vi "Start Live View.vi"(8 "error in (no error)":errorcluster, 10 "Camera State In":T3 {"Sub Region"."V Size"."Value" min=0 max=0 step=4; "Sub Region"."H Size"."Value" min=0 max=0 step=4; "Sub Region"."V Offset"."Value" min=0 max=0 step=4; "Sub Region"."H Offset"."Value" min=0 max=0 step=4}, 11 "Acquisition Settings":T1={"Save?"=FALSE, "DCIMG Path"=path "E:/test2", "Filename"="test", "Total Frames"=15, "Sender"=enum."UI"}) -> (0 "error out":errorcluster {"code" format="%.0x"}, 1 "New Image Out":T2, 2 "Camera State Out":T3 {"Sub Region"."V Size"."Value" min=0 max=0 step=4; "Sub Region"."H Size"."Value" min=0 max=0 step=4; "Sub Region"."V Offset"."Value" min=0 max=0 step=4; "Sub Region"."H Offset"."Value" min=0 max=0 step=4})   [LabVIEW 2015, in "Camera.lvlib"]
uses:
  Camera.lvlib
  Camera State.ctl
  Camera Loop State.ctl
  <vilib>/Utility/miscctls.llb/LVMinMaxIncTypeDef.ctl
  Acquisition Settings.ctl
  Live View State.ctl
  <vilib>/vision/Image Controls.llb/IMAQ Image.ctl
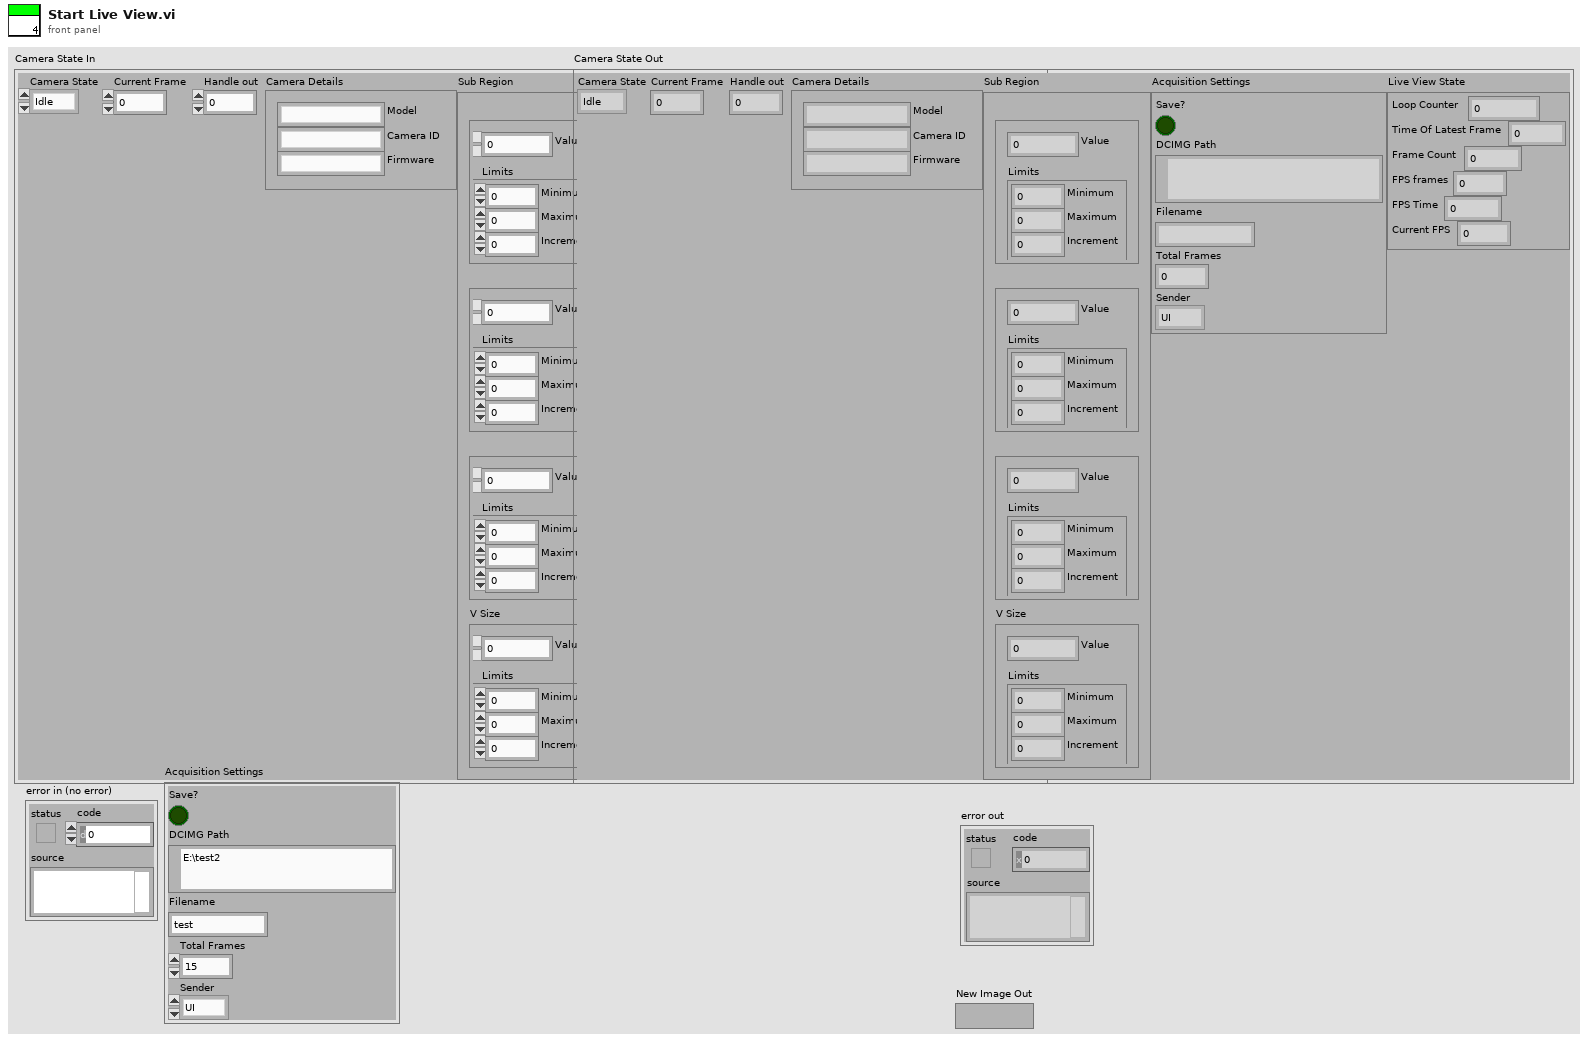
[diagram p1: front panel]
types:
  T1 = typedef "Camera.lvlib/Acquisition Settings.ctl" = cluster{"Save?":bool, "DCIMG Path":path, "Filename":string, "Total Frames":i32, "Sender":enum16{"UI", "Automation"}}
  T2 = typedef "IMAQ Image.ctl" = refnum<image>
  T3 = typedef "Camera.lvlib/Camera State.ctl" = cluster{"Camera State":T4, "Current Frame":i32, "Handle out":u32, "Camera Details":cluster{"Model":string, "Camera ID":string, "Firmware":string}, "Sub Region":cluster{"H Offset":cluster{"Value":i32, "Limits":T5}, "V Offset":cluster{"Value":i32, "Limits":T5}, "H Size":cluster{"Value":i32, "Limits":T5}, "V Size":cluster{"Value":i32, "Limits":T5}}, "Acquisition Settings":T1, "Live View State":T6}
  T4 = typedef "Camera.lvlib/Camera Loop State.ctl" = enum16{"Idle", "Live View", "Ready", "Acquiring"}
  T5 = typedef "LVMinMaxIncTypeDef.ctl" = cluster{"Minimum":dbl, "Maximum":dbl, "Increment":dbl}
  T6 = typedef "Camera.lvlib/Live View State.ctl" = cluster{"Loop Counter":i32, "Time Of Latest Frame":u32, "Frame Count":u32, "FPS frames":dbl, "FPS Time":u32, "Current FPS":dbl}
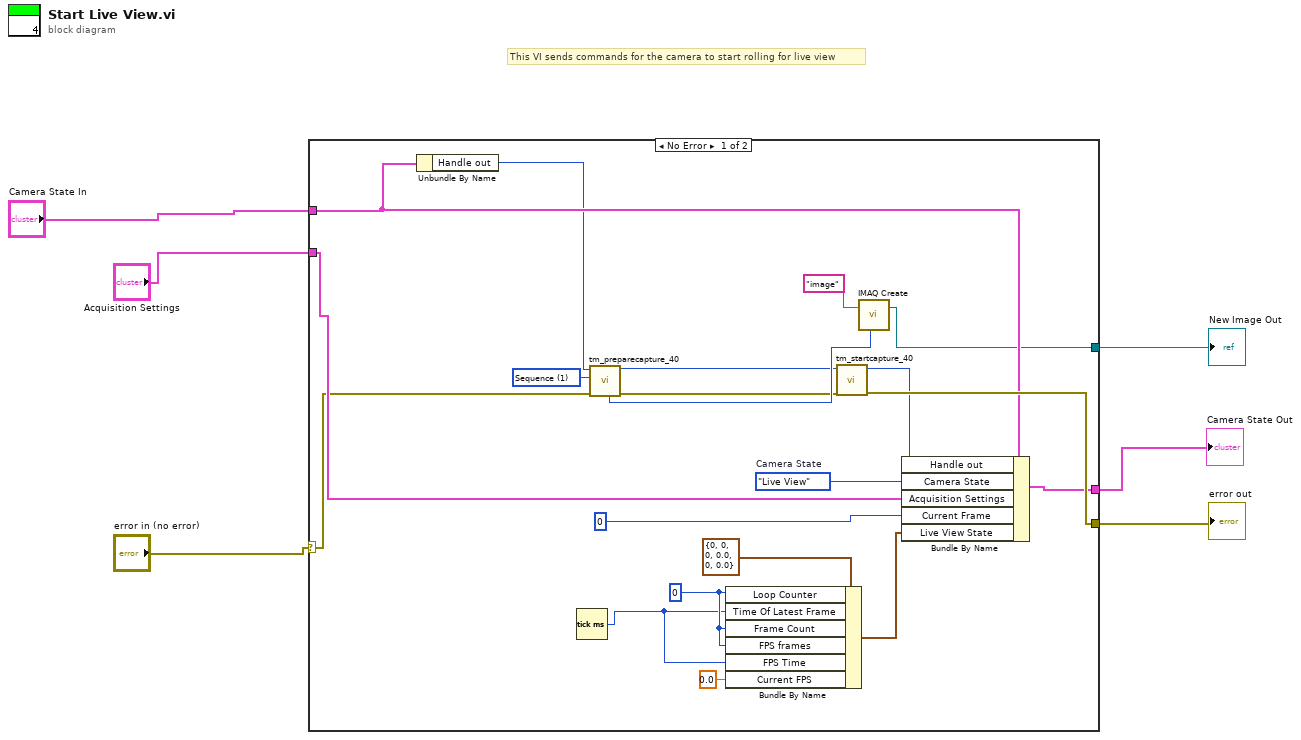
[diagram p0: block diagram]
diagram:
  # "This VI sends commands for the camera to start rolling for live view"
  n1 = case shown="No Error" "error in (no error)" {
    selector: "error in (no error)" -> [w17 w28]
    tunnel: [w24 w28] -> w6
    tunnel: "Camera State In" -> [w20 w27]
    tunnel: [w21 w27] -> w4
    tunnel: [w19 _] -> w2
    tunnel: "Acquisition Settings" -> [w18 _]
    frame No Error {
      w9 = 0 ("Loop Counter")
      w15 = 1 items=["Snap", "Sequence"] ("Capture mode")
      w26 = Camera_Loop_State."Live View"  # Camera State
      n2 = Unbundle By Name(w20) -> ("Handle out"=w16:u32)
      n3 = Tick Count (ms)() -> (millisecond timer value=w8:u32)
      n4 = call <userlib>:"tm_preparecapture_40.vi"("error in (no error)"=w17, "Capture mode"=w15, "Handle in"=w16) -> ("error out"=w12:errorcluster, "Handle out"=w13:u32, "Image type"=w14:u32)  [unwired: 5 in, 1 out]
      n5 = Bundle By Name(cluster=T6 {"Loop Counter"=0, "Time Of Latest Frame"=0, "Frame Count"=0, "FPS frames"=0.0, "FPS Time"=0, "Current FPS"=0.0} ("Live View State"), "Loop Counter"=w9, "Time Of Latest Frame"=w8, "Frame Count"=w9, "FPS frames"=w9, "FPS Time"=w8, "Current FPS"=0.0) -> (w11:T6)
      n6 = call <userlib>:"tm_startcapture_40.vi"("error in (no error)"=w12, "Handle in"=w13) -> ("error out"=w24:errorcluster, "Handle out"=w23:u32)  [unwired: 8 in]
      n7 = call "IMAQ Create"("Image Name"="image", "Image Type"=w14) -> ("New Image"=w19:T2)  [unwired: 3 in, 1 out]
      n8 = Bundle By Name(cluster=w20, "Handle out"=w23, "Camera State"=w26, "Acquisition Settings"=w18, "Current Frame"=0, "Live View State"=w11) -> (w21:T3)
    }
    frame Error {
    }
  }
  "Camera State Out" <- w4
  "error out" <- w6
  "New Image Out" <- w2
